vi "Measurements.vi"(8 "error in (no error)":errorcluster, 10 "BaseMeasurements":T1, 11 "Module":refnum<class "ModuleAdmin.lvclass">) -> (0 "error out":errorcluster)   [LabVIEW 2018, in "AcPwrModule.lvlib"]
uses:
  AcPwrModule.lvlib
  <userlib>/NIST/ModuleAdminLib/ModuleAdmin/ModuleAdmin.lvclass
  AcPwrPlugins/AcPwrBaseClass/TypeDefs/BaseMeasurements.ctl
  AcPwrPlugins/AcPwrBaseClass/TypeDefs/MeasType.ctl
  clEventType.ctl
  AcPwrPlugins/AcPwrBaseClass/AcPwrBase.lvclass
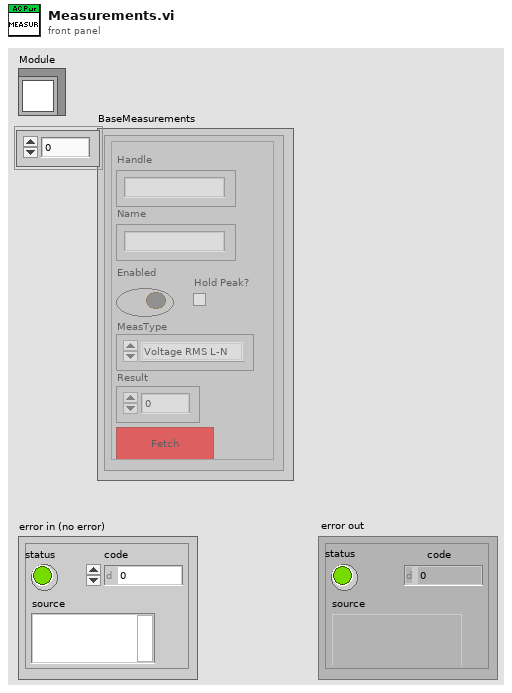
[diagram p1: front panel]
types:
  T1 = typedef "AcPwrPlugins.lvlib/AcPwrBase.lvclass/BaseMeasurements.ctl" = cluster{"Handle":string, "Name":string, "Enabled":bool, "Result":dbl, "MeasType":T2, "btnMeasFetch":bool, "Hold Peak?":bool}[]
  T2 = typedef "AcPwrPlugins.lvlib/AcPwrBase.lvclass/MeasType.ctl" = enum16{"Voltage RMS L-N", "Current RMS", "Frequency", "Voltage DC", "Current DC", "Power Factor", "Current Peak", "Power VA", "Real Power", "Voltage THD", "Voltage EHD", "Voltage OHD", "Current THD", "Current EHD", "Current OHD", "Voltage RMS L-L", "Phase Angle", "Power DC", "Crest Factor"}
  T3 = typedef "AcPwrModule.lvlib/clBroadcastEvents.ctl" = cluster{"DidInit":refnum<user-event>, "StatusUpdate":refnum<user-event>, "ErrorReport":refnum<user-event>, "DidStop":refnum<user-event>, "PathToINI":refnum<user-event>, "Measurements":refnum<user-event>, "LoadConfigFile":refnum<user-event>}
  T4 = typedef "AcPwrModule.lvlib/clEventType.ctl" = cluster{"ModuleID":i32, "Data":variant}
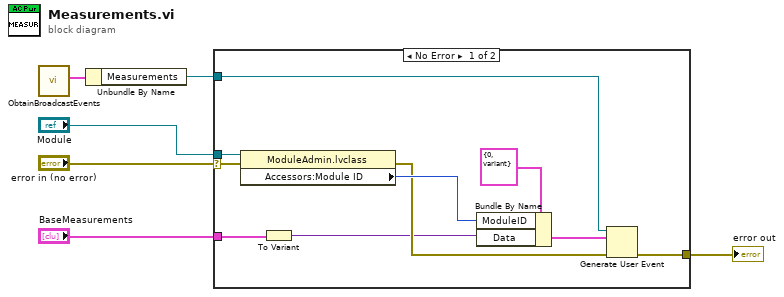
[diagram p0: block diagram]
diagram:
  n1 = call "ObtainBroadcastEvents.vi"() -> ("clAcPwrEvents"=w3:T3)  [unwired: 10 in, 1 out]
  n2 = Unbundle By Name(w3) -> ("Measurements"=w2:refnum<user-event>)
  n3 = case shown="No Error" "error in (no error)" {
    selector: "error in (no error)" -> [w16 w17]
    tunnel: "Module" -> [w15 _]
    tunnel: [w11 w17] -> w4
    tunnel: w2 -> [w10 _]
    tunnel: "BaseMeasurements" -> [w8 _]
    frame No Error {
      n4 = property class="ModuleAdmin.lvclass"(reference=w15, error in=w16) -> (error out=w13:errorcluster, "Accessors:Module ID"=w14:i32)  [unwired: 1 out]
      n5 = To Variant(anything=w8) -> (Variant=w7:variant)
      n6 = Bundle By Name(cluster=T4 {"ModuleID"=0, "Data"=variant} ("clEventType"), "ModuleID"=w14, "Data"=w7) -> (w9:T4)
      n7 = Generate User Event(user event=w10, event data cluster=w9, error in=w13) -> (error out=w11:errorcluster)  [unwired: 1 in, 1 out]
    }
    frame Error {
    }
  }
  "error out" <- w4
